vi "Read BehaviorPK.vi"(8 "error in (no error)":errorcluster, 11 "BehaviorData in":refnum<class "BehaviorData.lvclass">) -> (0 "error out":errorcluster, 2 "BehaviorPK":T1, 3 "BehaviorData out":refnum<class "BehaviorData.lvclass">)   [LabVIEW 2014, in "BehaviorData.lvclass"]
uses:
  BehaviorData.lvclass
  Database/BehPrimary.ctl
  BehaviorData.lvclass/BehaviorData.ctl
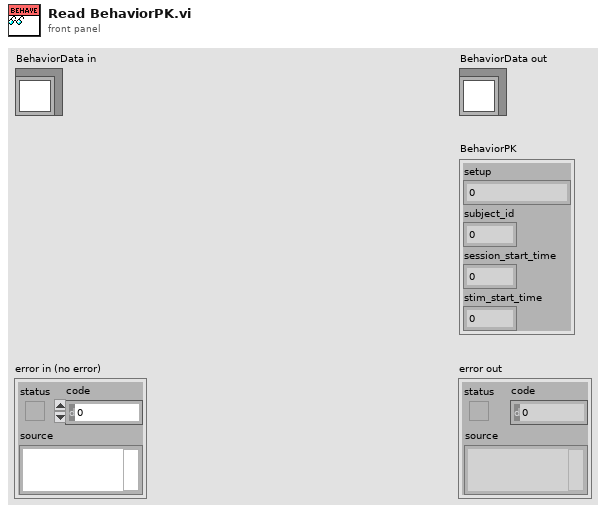
[diagram p1: front panel]
types:
  T1 = typedef "BehPrimary.ctl" = cluster{"setup":u8, "subject_id":i32, "session_start_time":dbl, "stim_start_time":dbl}
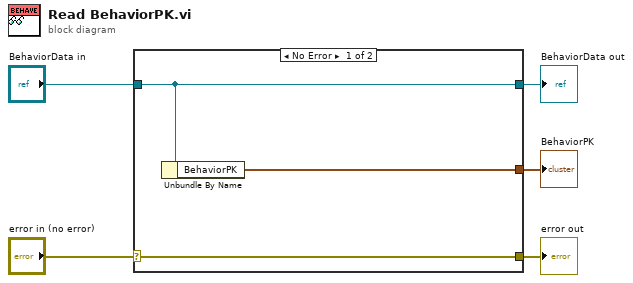
[diagram p0: block diagram]
diagram:
  n1 = case shown="No Error" "error in (no error)" {
    selector: "error in (no error)" -> [w8 w9]
    tunnel: [w8 w9] -> w4
    tunnel: [w7 w10] -> w2
    tunnel: "BehaviorData in" -> [w7 w10]
    tunnel: [w6 _] -> w1
    frame No Error {
      n2 = Unbundle By Name(w7) -> ("BehaviorPK"=w6:T1)
    }
    frame Error {
    }
  }
  "error out" <- w4
  "BehaviorData out" <- w2
  "BehaviorPK" <- w1
